vi "Construct Theme.vi"(4 "input":T1={"Text.Font Name"="Segoe UI", "Text.Font Size"=30, "Color"=0, "Text.Justification"=enum."Center", "messge color"={"border"=16777215, "fill"=16777215}}, 6 "message font":T1={"Text.Font Name"="Segoe UI", "Text.Font Size"=30, "Color"=0, "Text.Justification"=enum."Center", "messge color"={"border"=16777215, "fill"=16777215}}, 8 "error in (no error)":errorcluster, 9 "button colors":T2={"false color"={"border"=13816530, "fill"=16777215}, "hover color"={"border"=0, "fill"=0}, "press color"={"border"=1067897, "fill"=1067897}, "Boolean Text"=1668818, "Text.Font Name"="Segoe UI", "Text.Font Size"=20, "Bold?"=TRUE, "Itallic?"=FALSE}, 10 "dialog colors":T3={"Header"=1668818, "Background"=1668818, "Picture Background"=16777216}) -> (0 "error out":errorcluster, 3 "Theme out":refnum<class "Theme.lvclass">)   [LabVIEW 2021, in "Theme.lvclass"]
doc: "Construct a theme object from an input of all of the type defs\n\n<b>Code Developed By:</b>\nTechnology Service Corporation\n1983 S Liberty Drive\nBloomington, IN 47403\nPhone: 812 558-7100\nwww.tsc.com/atcs\n\nDeveloper:\nDaniel Coons"
uses:
  Theme.lvclass
  Dialog colors--typedef.ctl
  Button colors--typedef.ctl
  message box--typdef.ctl
  Theme.lvclass/Theme.ctl
  Popup/PopUp Theme Global.vi
  Popup/Popup.lvclass
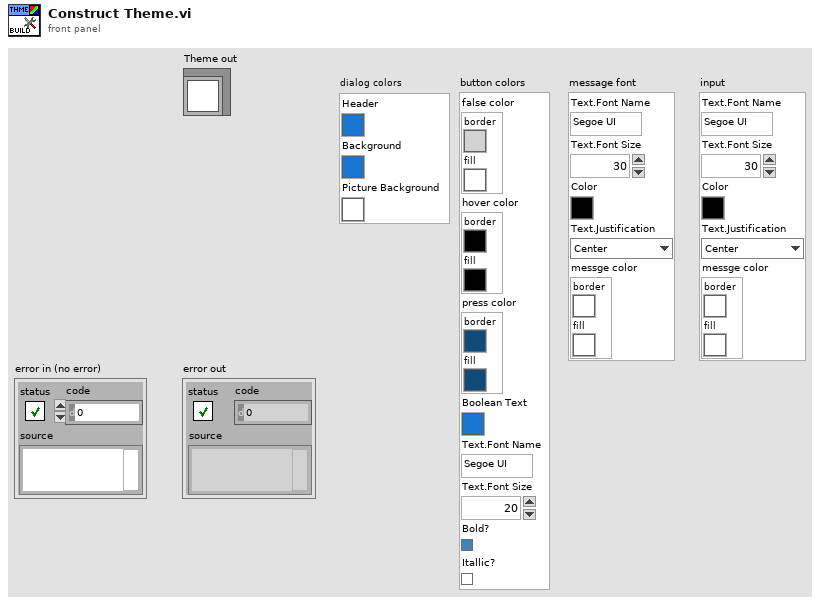
[diagram p1: front panel]
types:
  T1 = typedef "Theme.lvclass/message box--typdef.ctl" = cluster{"Text.Font Name":string, "Text.Font Size":u32, "Color":u32, "Text.Justification":enum16{"Left", "Center", "Right"}, "messge color":cluster{"border":u32, "fill":u32}}
  T2 = typedef "Theme.lvclass/Button colors--typedef.ctl" = cluster{"false color":cluster{"border":u32, "fill":u32}, "hover color":cluster{"border":u32, "fill":u32}, "press color":cluster{"border":u32, "fill":u32}, "Boolean Text":u32, "Text.Font Name":string, "Text.Font Size":u32, "Bold?":bool, "Itallic?":bool}
  T3 = typedef "Theme.lvclass/Dialog colors--typedef.ctl" = cluster{"Header":u32, "Background":u32, "Picture Background":u32}
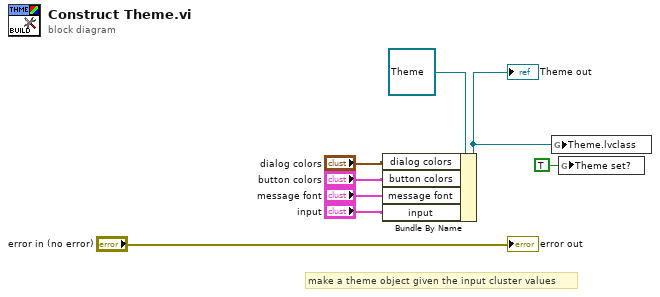
[diagram p0: block diagram]
diagram:
  # "make a theme object given the input cluster values"
  n1 = Bundle By Name(cluster=refnum<class "Theme.lvclass"> refnum ("Theme.lvclass"), "dialog colors"="dialog colors", "button colors"="button colors", "message font"="message font", "input"="input") -> (w2:refnum<class "Theme.lvclass">)
  "Theme out" <- w2
  n2 = global write "PopUp Theme Global.vi" "Theme.lvclass"(w2) -> ()
  n3 = global write "PopUp Theme Global.vi" "Theme set?"(TRUE ("Theme set?")) -> ()
  "error out" <- "error in (no error)"
